vi "Set IConfiguration.vi"(10 "IConfiguration":refnum<class "IConfiguration.lvclass">, 11 "gRPC XNET Read Raw CAN Frame Strategy in":refnum<class "gRPC XNET Read Raw CAN Frame Strategy.lvclass">) -> (3 "gRPC XNET Read Raw CAN Frame Strategy out":refnum<class "gRPC XNET Read Raw CAN Frame Strategy.lvclass">)   [LabVIEW 2024, in "gRPC XNET Read Raw CAN Frame Strategy.lvclass"]
uses:
  gRPC XNET Read Raw CAN Frame Strategy.lvclass
  Source/Interfaces/IConfiguration/IConfiguration.lvclass
  gRPC XNET Read Raw CAN Frame Strategy.lvclass/gRPC XNET Read Raw CAN Frame Strategy.ctl
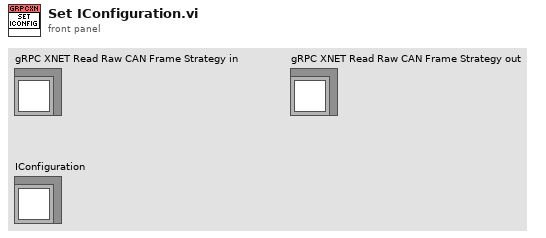
[diagram p1: front panel]
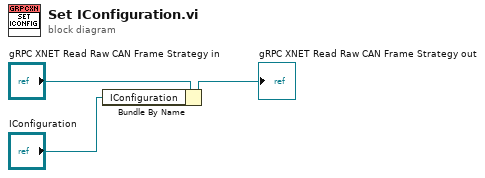
[diagram p0: block diagram]
diagram:
  n1 = Bundle By Name(cluster="gRPC XNET Read Raw CAN Frame Strategy in", "IConfiguration"="IConfiguration") -> (→"gRPC XNET Read Raw CAN Frame Strategy out":refnum<class "gRPC XNET Read Raw CAN Frame Strategy.lvclass">)
